vi "auto sensitivity(SubVI).vi"(8 "量程":enum16{"量程每次测量会判定", "量程不变为设定值"}(ring), 9 "abort":refnum<queue>, 10 "量程初始":i32, 11 "VISA引用句柄输入":refnum<visa-resource-name>) -> (0 "error out":errorcluster, 1 "量程结束":i32, 2 "VISA引用句柄输出":refnum<visa-resource-name>)   [LabVIEW 2019, in "SubVI.lvlib"]
uses:
  SubVI.lvlib
  lib/Stanford Research 830/Stanford Research 830.lvlib
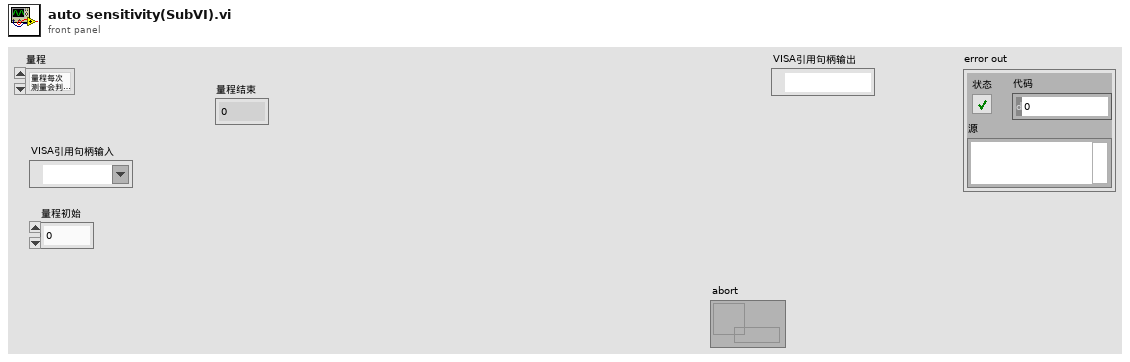
[diagram p1: front panel]
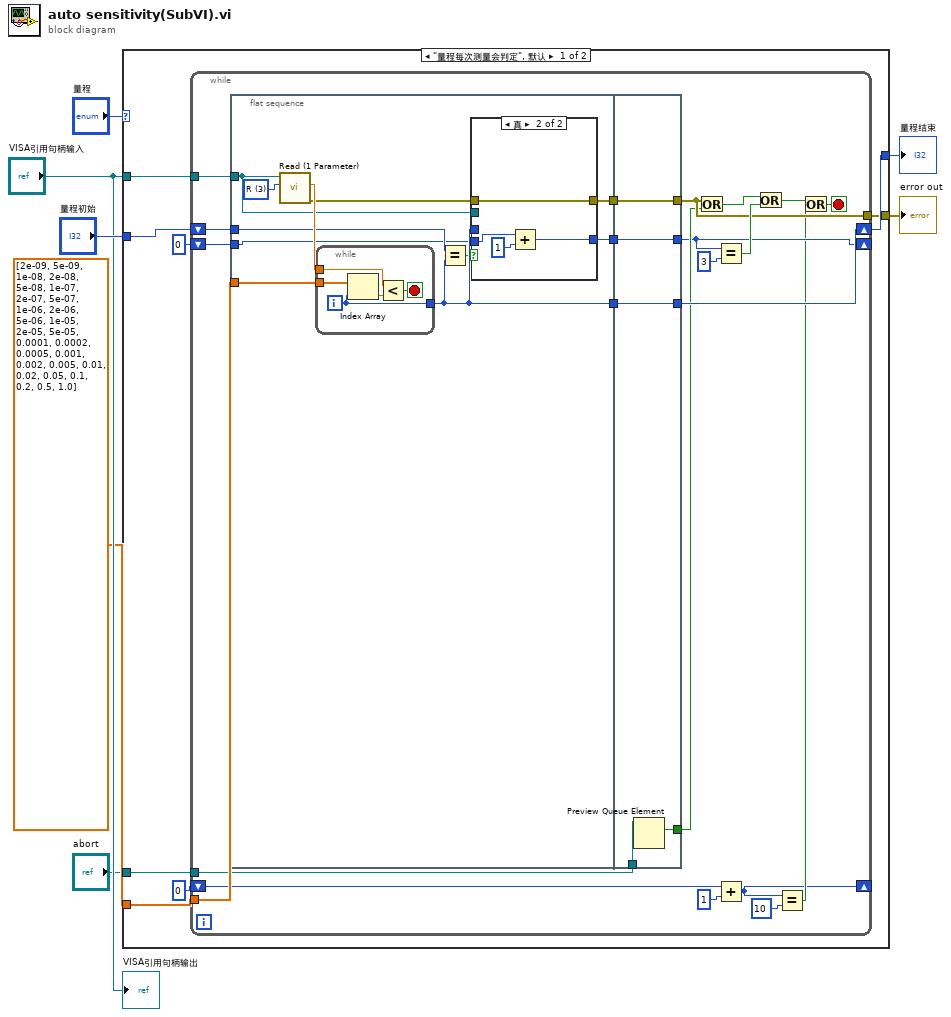
[diagram p0: block diagram]
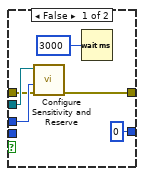
[diagram p2: hidden frame]
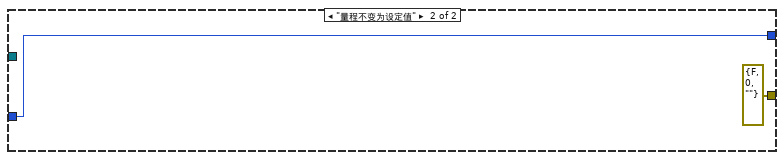
[diagram p3: hidden frame]
diagram:
  n1 = case shown="\"量程每次测量会判定\", 默认" "量程" {
    tunnel: [w15 w70] -> w7
    tunnel: "量程初始" -> [w14 w70]
    tunnel: "VISA引用句柄输入" -> [w13 _]
    tunnel: dbl[] [2e-09, 5e-09, 1e-08, 2e-08, 5e-08, 1e-07, 2e-07, 5e-07, 1e-06, 2e-06, 5e-06, 1e-05, 2e-05, 5e-05, 0.0001, 0.0002, 0.0005, 0.001, 0.002, 0.005, 0.01, 0.02, 0.05, 0.1, 0.2, 0.5, 1.0] -> [w12 _]
    tunnel: "abort" -> [w10 _]
    tunnel: [w9 errorcluster {"status"=FALSE, "code"=0, "source"=""} ("error out")] -> w1
    frame "量程每次测量会判定", Default {
      n2 = while {
        tunnel: w13 -> [w37]
        tunnel: w12 -> [w36]
        shift-right: [w34] -> w15
        shift-left: w14 -> [w33]
        shift-right: [w23] -> _
        shift-left: 0 -> [w32]
        tunnel: w10 -> [w27]
        tunnel: [w26] -> w9
        shift-right: [w16] -> _
        shift-left: 0 -> [w18]
        stop <- w19 stop-if-true
        n3 = flat-sequence {
          tunnel: w32 -> [w42]
          tunnel: w33 -> [w43]
          tunnel: w36 -> [w46]
          tunnel: w37 -> [w40]
          tunnel: [w41] -> w30
          tunnel: [w48] -> w29
          tunnel: [w38] -> w28
          tunnel: [w66] -> w26
          tunnel: [w67] -> w34
          tunnel: [w68] -> w23
          tunnel: w30 -> [w68]
          tunnel: w29 -> [w67]
          tunnel: w28 -> [w66]
          tunnel: w27 -> [w65]
          tunnel: [w64] -> w25
          frame #0 {
            w45 = u16 3 items=["X"=1, "Y"=2, "R"=3, "Theta"=4, "Channel 1"=5, "Channel 2"=6, "Aux In 1"=7, "Aux In 2"=8, "Aux In 3"=9, "Aux In 4"=10] ("Parameter (1: X)")
            n4 = call "Read (1 Parameter).vi"("Parameter (1: X)"=w45, "VISA resource name"=w40) -> ("error out"=w39:errorcluster, "Measurement"=w44:dbl)  [unwired: 7 in, 1 out]
            n5 = while {
              tunnel: [w51] -> w48
              tunnel: w46 -> [w50]
              tunnel: w44 -> [w49]
              i -> [w51]
              stop <- w53 stop-if-true
              n6 = Index Array(array=w50, index=w51) -> (element=w52:dbl)
              n7 = Less?(x=w49, y=w52) -> (x < y?=w53:bool)
            }
            n8 = Equal?(x=w43, y=w48) -> (x = y?=w47:bool)
            n9 = case shown="真" w47 {
              tunnel: w48 -> [w59 _]
              tunnel: w40 -> [w58 _]
              tunnel: w42 -> [_ w62]
              tunnel: [0 w61] -> w41
              tunnel: w39 -> [w55 w60]
              tunnel: [w54 w60] -> w38
              frame False {
                n10 = call "Configure Sensitivity and Reserve.vi"("error in (no error)"=w55, "Sensitivity (-1: Auto gain)"=w59, "VISA resource name"=w58) -> ("error out"=w54:errorcluster)  [unwired: 7 in, 1 out]
                n11 = Wait (ms)(milliseconds to wait=u32 3000 ("等待时间（毫秒）")) -> ()  [unwired: 1 out]
              }
              frame True {
                n12 = Add(x=w62, y=1) -> (x+y=w61:i32)
              }
            }
          }
          frame #1 {
            n13 = Preview Queue Element(queue=w65) -> (element=w64:bool)  [unwired: 2 in, 3 out]
          }
        }
        n14 = Or(x=w26, y=w25) -> (x .or. y?=w24:bool)
        n15 = Equal?(x=w23, y=3) -> (x = y?=w31:bool)
        n16 = Add(x=w18, y=1) -> (x+y=w16:i32)
        n17 = Or(x=w24, y=w31) -> (x .or. y?=w21:bool)
        n18 = Equal?(x=w16, y=10) -> (x = y?=w20:bool)
        n19 = Or(x=w21, y=w20) -> (x .or. y?=w19:bool)
      }
    }
    frame "量程不变为设定值" {
    }
  }
  "量程结束" <- w7
  "error out" <- w1
  "VISA引用句柄输出" <- "VISA引用句柄输入"
